vi "Generate Event.vi"(8 "Error In":errorcluster, 9 "Event Data":refnum<class "Event Data.lvclass">, 10 "Event Name":string, 11 "Event Source In":refnum<class "Event Source.lvclass">) -> (0 "Error Out":errorcluster, 3 "Event Source Out":refnum<class "Event Source.lvclass">)   [LabVIEW 2020, in "Event Source.lvlib" / "Event Source.lvclass"]
doc: "This method generates/fires the Event wired to the input. Firing an event looks up all actors who Registered to listen to this Event and sends to them this Event on a Zero Coupling based message defined during Registration. Errors on broadcasting the event i.e. enqueuer of the registrant not existing, are ignored.\n\n<b>IMPORTANT</b> - Only call this method within actor core of your Event Source Actor. From helper loops call the Send Generate Event message to self. This is to make sure your actor works with all registered listeners."
uses:
  Event Source.lvclass
  Event Data/Event Data.lvclass
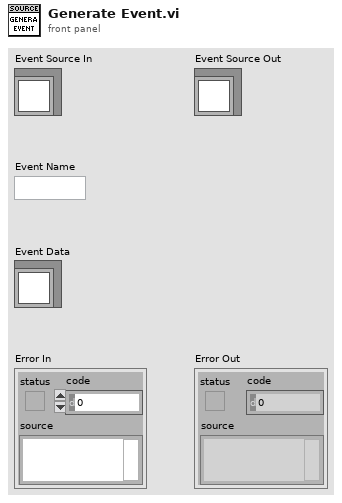
[diagram p1: front panel]
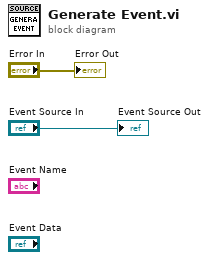
[diagram p0: block diagram]
diagram:
  "Error Out" <- "Error In"
  "Event Source Out" <- "Event Source In"
